vi "Main.vi"(11 "Module Admin":refnum<class "Delacor_lib_QMH_Cloneable Module Admin.lvclass">) -> ()   [LabVIEW 2025, in "Stepper.lvlib"]
doc: "This template is based off of the Queued Message Handler design pattern and the Queued Message Handler project template that ships with LabVIEW.\n\nThe main difference is that the queue is private to this module and communication between modules is performed via Broadcast and Request events.\n\nRequest events are wrapped in public API methods and are handled in the Event Handling Loop (EHL) of this VI. Any module can register for Broadcast events sent by this module. The EHL generates messages based on user interface actions.\n\nThe Message Handling Loop (MHL) processes messages generated by the EHL, or by other messages. The messages are string values, so new messages can be added easily to the Message Cases case structure in the MHL. Each message cluster can also provide an optional value for Message Data, which is a variant that can be converted to whatever message-specific data is required.\n_____\nBased on DQMH Dev Tools: Project Template 7.1.2.1547."
uses:
  Stepper.lvlib
  <vilib>/Delacor/Delacor QMH/Libraries/Cloneable Module Admin_class/Delacor_lib_QMH_Cloneable Module Admin.lvclass
  C:/Program Files/National Instruments/LabVIEW 2025/vi.lib/Delacor/Delacor QMH/Libraries/Module Admin_class/Delacor_lib_QMH_Module Admin.lvclass
  Module Data--cluster.ctl
  Classes/Stepper/Stepper.lvclass
  <vilib>/Delacor/Delacor QMH/Libraries/Message Queue_class/Delacor_lib_QMH_Message Queue.lvclass/Delacor_lib_QMH_Message Queue.ctl
  <vilib>/Delacor/Delacor QMH/Libraries/Cloneable Module Admin_class/Delacor_lib_QMH_Cloneable Module Admin.lvclass/Delacor_lib_QMH_Cloneable Module Admin.ctl
  Stop Argument--cluster.ctl
  <vilib>/Delacor/Delacor QMH/Libraries/Module Admin_class/Delacor_lib_QMH_Module Admin.lvclass/Delacor_lib_QMH_Module Admin.ctl
  close Argument--cluster.ctl
  close (Reply Payload)--cluster.ctl
  init driver Argument--cluster.ctl
  init driver (Reply Payload)--cluster.ctl
  Clear Motor Error Argument--cluster.ctl
  Clear Motor Error (Reply Payload)--cluster.ctl
  read config Argument--cluster.ctl
  read config (Reply Payload)--cluster.ctl
  Read Angle Argument--cluster.ctl
  Read Angle (Reply Payload)--cluster.ctl
  Jog Argument--cluster.ctl
  Jog (Reply Payload)--cluster.ctl
  Go To Angle Argument--cluster.ctl
  Go To Angle (Reply Payload)--cluster.ctl
  <vilib>/Utility/miscctls.llb/LVPointTypeDef.ctl
  <vilib>/Delacor/Delacor QMH/Libraries/Message Queue_class/Delacor_lib_QMH_Enqueue Message (Single).vi
  <vilib>/Delacor/Delacor QMH/Libraries/Cloneable Module Admin_class/Delacor_lib_QMH_Get Module ID.vi
  <vilib>/Delacor/Delacor QMH/Libraries/Module Admin_class/Delacor_lib_QMH_Get External Launch.vi
  <vilib>/Delacor/Delacor QMH/Libraries/Message Queue_class/Delacor_lib_QMH_Message Queue.lvclass
panel:
  out "error out":errorcluster
  out "Status":string
  in  "Simulate EHL Error":bool
  in  "Simulate MHL Error":bool
  # "Other processes communicate with this Module via its Public API (wrappers for its Request Events).\n\nThis Module communicates with other processes via its Broadcast Events.\nAny process that wants to receive these messages can register for this module's Broadcast events."
  # "This template is for the DQMH framework. See the block diagram for more information on how to use this template."
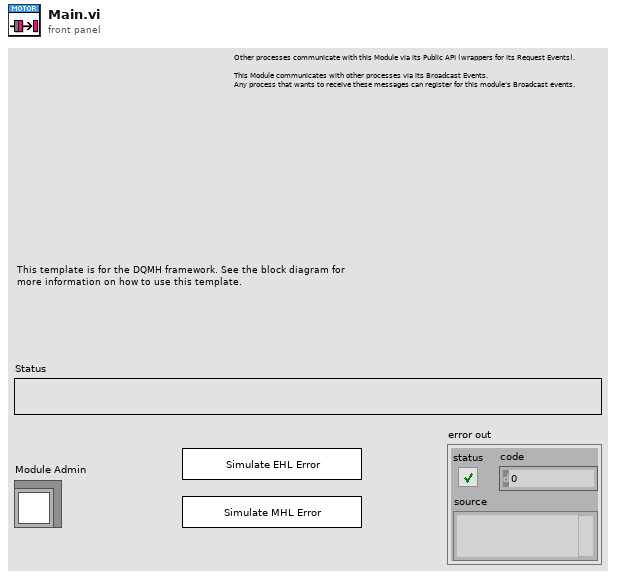
[diagram p1: front panel]
types:
  T1 = typedef "Stepper.lvlib/Request Events--cluster.ctl" = cluster{"Stop Module":refnum<user-event>, "Show Panel":refnum<user-event>, "Hide Panel":refnum<user-event>, "Show Diagram":refnum<user-event>, "Get Module Execution Status":refnum<user-event>, "close":refnum<user-event>, "init":refnum<user-event>, "init driver":refnum<user-event>, "Clear Motor Error":refnum<user-event>, "read config":refnum<user-event>, "Read Angle":refnum<user-event>, "Jog":refnum<user-event>, "Go To Angle":refnum<user-event>}
  T2 = typedef "Stepper.lvlib/Module Data--cluster.ctl" = cluster{"Status":string, "Stepper":refnum<class "Stepper.lvclass">}
  T3 = enum32{"invalid lock state", "Not Locked", "Locked (No Password)", "Password-protected"}
  T4 = typedef "Stepper.lvlib/Stop Argument--cluster.ctl" = cluster{"Module ID":i32, "Origin":string, "Exit via Stop Module Req?":bool, "Wait for Module to stop?":bool}
  T5 = typedef "Stepper.lvlib/close Argument--cluster.ctl" = cluster{"Module ID":i32, "Wait Notifier":refnum<notifier>, "wait for reply":bool}
  T6 = typedef "Stepper.lvlib/init driver Argument--cluster.ctl" = cluster{"Module ID":i32, "Wait Notifier":refnum<notifier>, "wait for reply":bool}
  T7 = typedef "Stepper.lvlib/Clear Motor Error Argument--cluster.ctl" = cluster{"Module ID":i32, "Wait Notifier":refnum<notifier>, "wait for reply":bool}
  T8 = typedef "Stepper.lvlib/read config Argument--cluster.ctl" = cluster{"Module ID":i32, "config file path":path, "Wait Notifier":refnum<notifier>, "wait for reply":bool}
  T9 = typedef "Stepper.lvlib/Read Angle Argument--cluster.ctl" = cluster{"Module ID":i32, "Wait Notifier":refnum<notifier>, "wait for reply":bool}
  T10 = typedef "Stepper.lvlib/Jog Argument--cluster.ctl" = cluster{"Module ID":i32, "CCW? (T)":bool, "[rpm]":u16, "Wait Notifier":refnum<notifier>, "wait for reply":bool}
  T11 = typedef "Stepper.lvlib/Go To Angle Argument--cluster.ctl" = cluster{"Module ID":i32, "Angle":dbl, "Velocity [rpm]":i32, "Pause Time [ms]":i32, "Wait Notifier":refnum<notifier>, "wait for reply":bool}
  T12 = typedef "LVPointTypeDef.ctl" = cluster{"Horizontal":i16, "Vertical":i16}
  T13 = enum32{"Invalid", "Standard", "Closed", "Hidden", "Minimized", "Maximized"}
  T14 = typedef "Stepper.lvlib/close (Reply Payload)--cluster.ctl" = cluster{"Module ID":i32, "error":errorcluster}
  T15 = typedef "Stepper.lvlib/init driver (Reply Payload)--cluster.ctl" = cluster{"Module ID":i32, "error":errorcluster}
  T16 = typedef "Stepper.lvlib/Clear Motor Error (Reply Payload)--cluster.ctl" = cluster{"Module ID":i32, "error":errorcluster}
  T17 = typedef "Stepper.lvlib/read config (Reply Payload)--cluster.ctl" = cluster{"Module ID":i32, "error":errorcluster}
  T18 = typedef "Stepper.lvlib/Read Angle (Reply Payload)--cluster.ctl" = cluster{"Module ID":i32, "Angle":dbl, "error":errorcluster}
  T19 = typedef "Stepper.lvlib/Jog (Reply Payload)--cluster.ctl" = cluster{"Module ID":i32, "Angle":dbl, "error":errorcluster}
  T20 = typedef "Stepper.lvlib/Go To Angle (Reply Payload)--cluster.ctl" = cluster{"Module ID":i32, "Angle":dbl, "error":errorcluster}
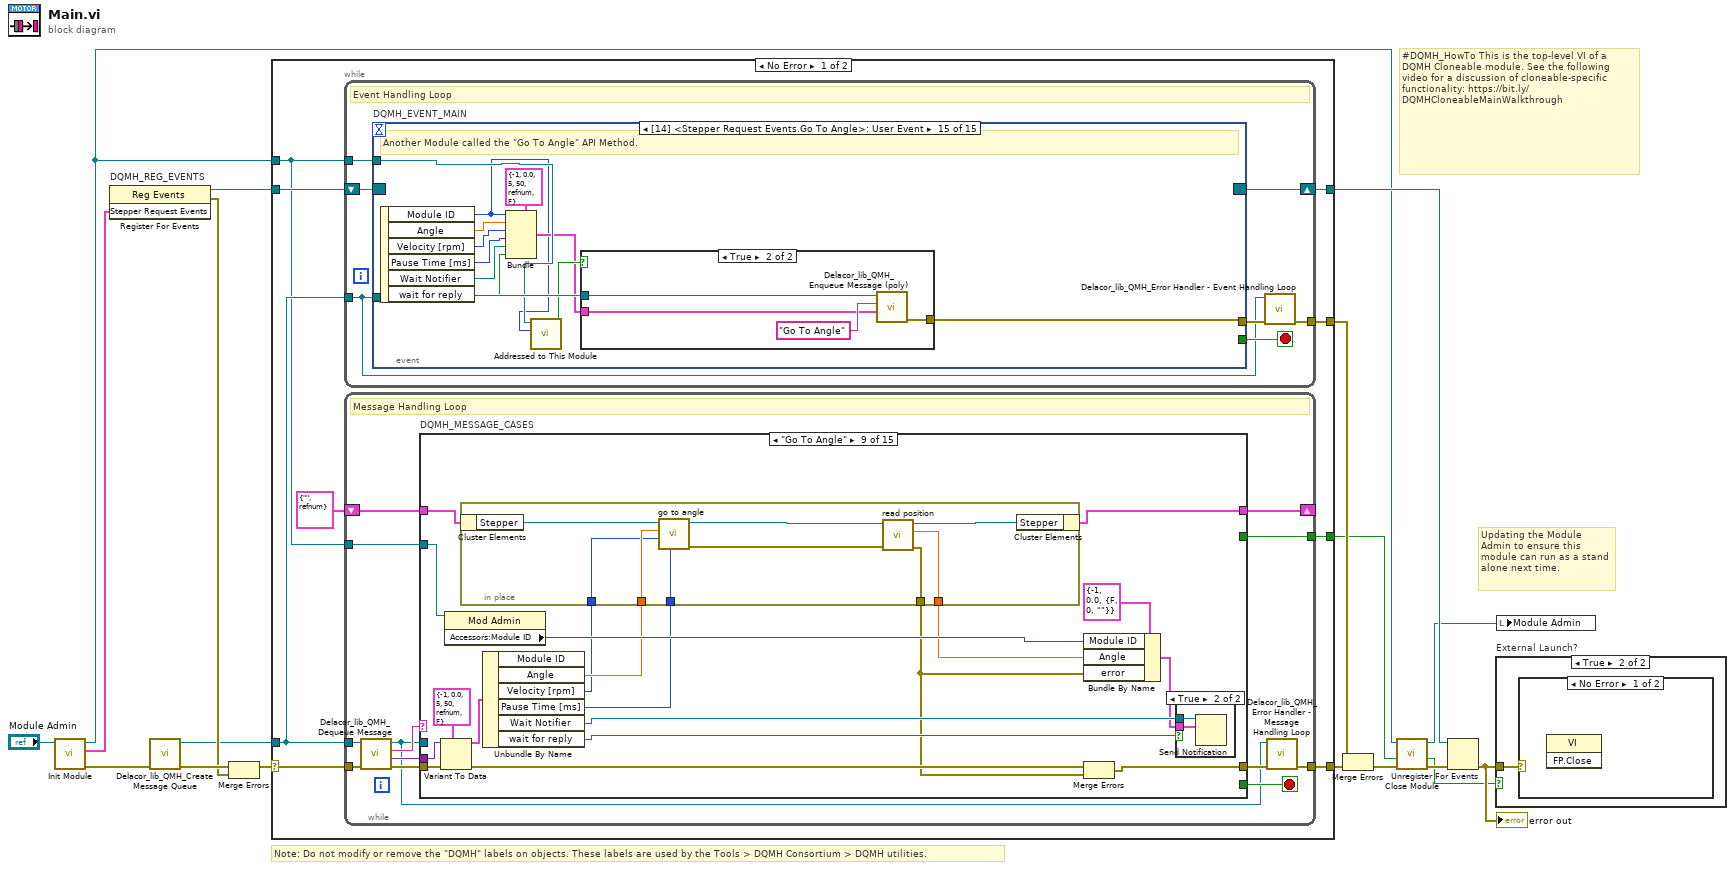
[diagram p0: block diagram]
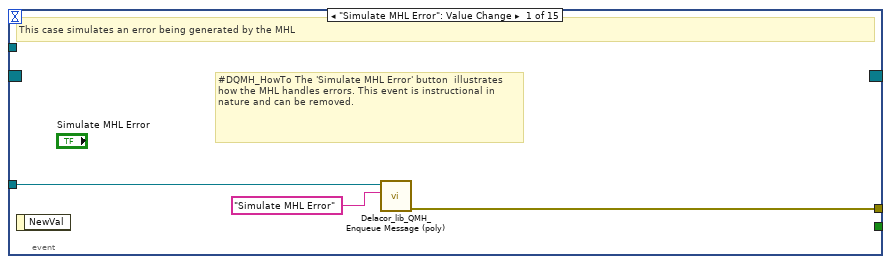
[diagram p2: hidden frame]
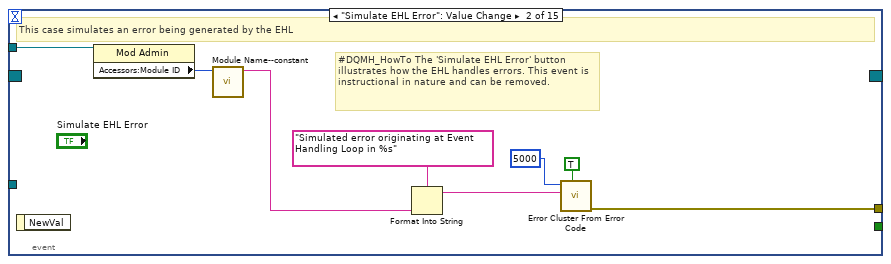
[diagram p3: hidden frame]
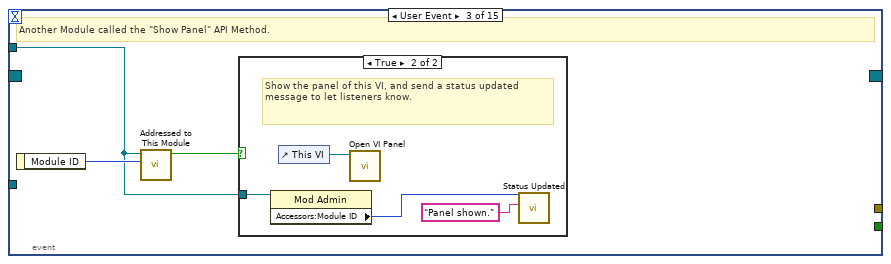
[diagram p4: hidden frame]
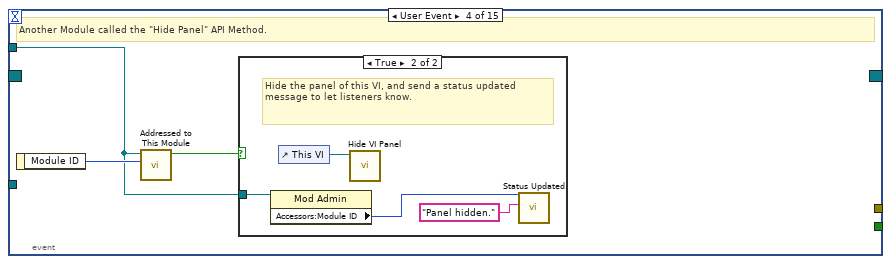
[diagram p6: hidden frame]
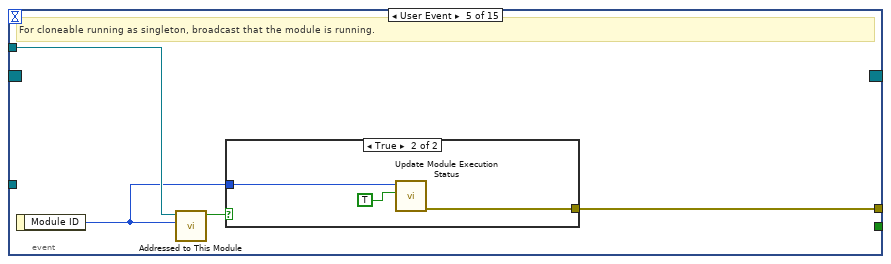
[diagram p8: hidden frame]
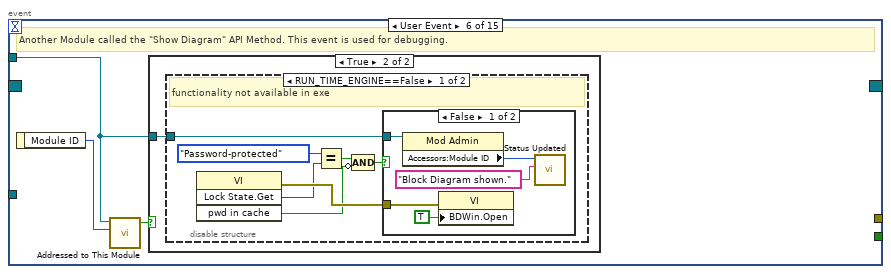
[diagram p10: hidden frame]
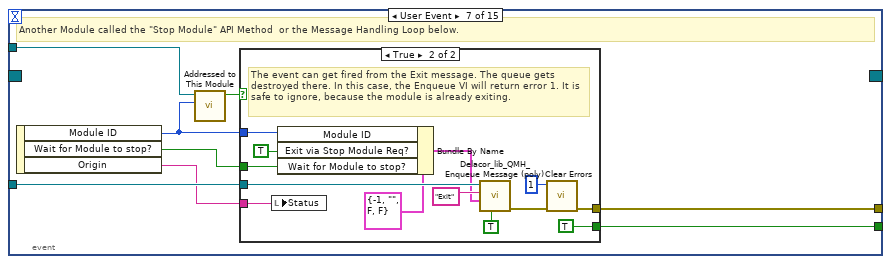
[diagram p14: hidden frame]
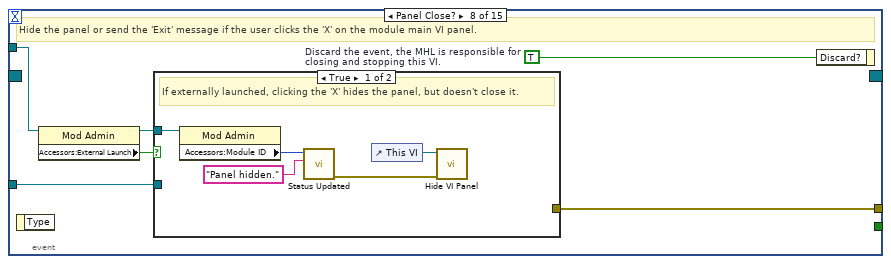
[diagram p16: hidden frame]
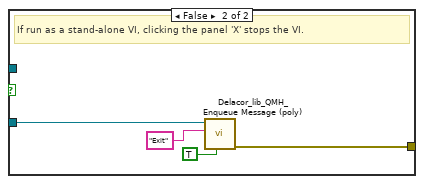
[diagram p17: hidden frame]
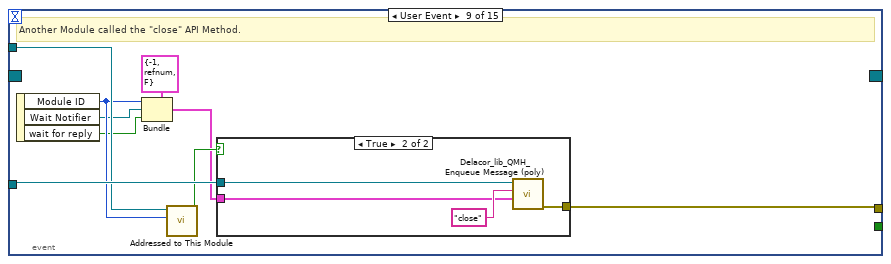
[diagram p18: hidden frame]
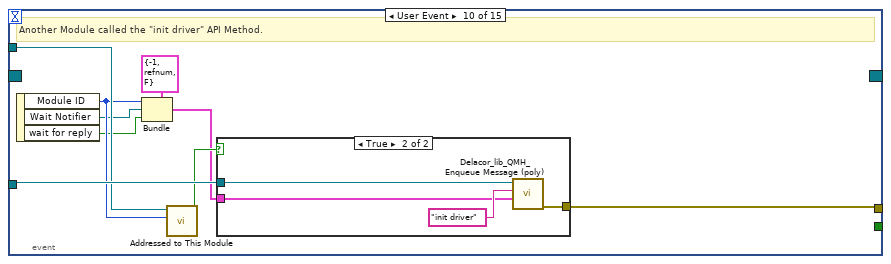
[diagram p20: hidden frame]
diagram:
  # "#DQMH_HowTo This is the top-level VI of a DQMH Cloneable module. See the following video for a discussion of cloneable-specific functionality: https://bit.ly/DQMHCloneableMainWalkthrough"
  # "Note: Do not modify or remove the \"DQMH\" labels on objects. These labels are used by the Tools > DQMH Consortium > DQMH utilities."
  # "Updating the Module Admin to ensure this module can run as a stand alone next time."
  n1 = call "Init Module.vi"("Cloneable Module Admin in"="Module Admin") -> ("error out"=w15:errorcluster, "Stepper Request Events"=w7:T1, "Cloneable Module Admin out"=w4:refnum<class "Delacor_lib_QMH_Cloneable Module Admin.lvclass">)  [unwired: 8 in]
  n2 = register-events "DQMH_REG_EVENTS"(w7) -> (reference out=w8:refnum<event-registration>, error out=w10:errorcluster)  [unwired: 2 in]
  n3 = call <vilib>:"Delacor_lib_QMH_Create Message Queue.vi"("error in"=w15) -> ("error out"=w12:errorcluster, "Message Queue"=w6:refnum<class "Delacor_lib_QMH_Message Queue.lvclass">)  [unwired: 9 in]
  n4 = Merge Errors(w12, w10) -> (w11:errorcluster)
  n5 = case shown="No Error" w11 {
    selector: w11 -> [w25 w489]
    tunnel: [w27 w488] -> w16
    tunnel: [w24 w487] -> w9
    tunnel: w8 -> [w22 w487]
    tunnel: w6 -> [w21 w480]
    tunnel: [w26 _] -> w17
    tunnel: w4 -> [w20 w483]
    tunnel: [w19 _] -> w2
    frame No Error {
      n6 = while {
        tunnel: w21 -> [w28]
        shift-right: [w31] -> w24
        shift-left: w22 -> [w32]
        tunnel: [w33] -> w26
        tunnel: w20 -> [w29]
        stop <- w30 stop-if-true
        # "Event Handling Loop"
        n7 = event "DQMH_EVENT_MAIN" shown="[14] <Stepper Request Events.Go To Angle>: User Event" {
          selector: w32 -> [_ _ _ _ _ _ _ _ _ _ _ _ _ _ _]
          dyn-events: [_ _ _ _ _ _ _ _ _ _ _ _ _ _ _] -> w31
          timeout: _ -> [_ _ _ _ _ _ _ _ _ _ _ _ _ _ _]
          tunnel: [_ _ _ _ _ _ w86 _ _ _ _ _ _ _ _] -> w30
          tunnel: w28 -> [w36 _ _ _ _ _ w89 w106 w127 w140 w153 w167 w180 w195 w211]
          tunnel: [w37 w45 _ _ w63 _ w90 w109 w119 w132 w145 w158 w172 w185 w200] -> w34
          tunnel: w29 -> [_ w44 w46 w53 w61 w67 w88 w107 w125 w138 w151 w165 w178 w193 w209]
          event "Simulate MHL Error": Value Change {
            # "#DQMH_HowTo The 'Simulate MHL Error' button  illustrates how the MHL handles errors. This event is instructional in nature and can be removed."
            # "This case simulates an error being generated by the MHL"
            n8 = event-data() -> ()  [unwired: 1 in, 1 out]
            n9 = call-poly <vilib>:"Delacor_lib_QMH_Enqueue Message (poly).vi"("Message"="Simulate MHL Error", "Message Queue in"=w36) -> ("error out"=w37:errorcluster)  [unwired: 8 in, 1 out]
          }
          event "Simulate EHL Error": Value Change {
            # "#DQMH_HowTo The 'Simulate EHL Error' button  illustrates how the EHL handles errors. This event is instructional in nature and can be removed."
            # "This case simulates an error being generated by the EHL"
            n10 = event-data() -> ()  [unwired: 1 in, 1 out]
            n11 = property on="Property Node" class="Mod Admin"(reference=w44) -> ("Accessors:Module ID"=w43:i32)  [unwired: 1 in, 2 out]
            n12 = call "Module Name--constant.vi"("Module ID"=w43) -> ("Module Name"=w38:string)  [unwired: 10 in]
            n13 = Format Into String(format string="Simulated error originating at Event Handling Loop in %s", w38) -> (resulting string=w41:string)  [unwired: 2 in, 1 out]
            n14 = call <vilib>:"Error Cluster From Error Code.vi"("show call chain? (False)"=TRUE, "error message (\"\")"=w41, "error code (0)"=5000) -> ("error out"=w45:errorcluster)  [unwired: 6 in]
          }
          event User Event {
            # "Another Module called the \"Show Panel\" API Method."
            n15 = event-data() -> ("Module ID"=w47:i32)  [unwired: 1 in]
            n16 = call "Addressed to This Module.vi"("Module ID from Argument"=w47, "Module Admin"=w46) -> ("Addressed to this instance?"=w48:bool)  [unwired: 8 in, 1 out]
            n17 = case shown="True" w48 {
              tunnel: w46 -> [_ w50]
              frame False {
              }
              frame True {
                # "Show the panel of this VI, and send a status updated message to let listeners know."
                n18 = property on="Property Node" class="Mod Admin"(reference=w50) -> ("Accessors:Module ID"=w49:i32)  [unwired: 1 in, 2 out]
                n19 = control-ref of="This VI"() -> (w52:refnum<vi>)
                n20 = call "Open VI Panel.vi"("VI"=w52) -> ()  [unwired: 10 in, 1 out]
                n21 = call "Status Updated.vi"("Status"="Panel shown." ("format string"), "Module ID"=w49) -> ()  [unwired: 9 in, 1 out]
              }
            }
          }
          event User Event {
            # "Another Module called the \"Hide Panel\" API Method."
            n22 = event-data() -> ("Module ID"=w54:i32)  [unwired: 1 in]
            n23 = call "Addressed to This Module.vi"("Module ID from Argument"=w54, "Module Admin"=w53) -> ("Addressed to this instance?"=w55:bool)  [unwired: 8 in, 1 out]
            n24 = case shown="True" w55 {
              tunnel: w53 -> [_ w57]
              frame False {
              }
              frame True {
                # "Hide the panel of this VI, and send a status updated message to let listeners know."
                n25 = property on="Property Node" class="Mod Admin"(reference=w57) -> ("Accessors:Module ID"=w56:i32)  [unwired: 1 in, 2 out]
                n26 = control-ref of="This VI"() -> (w59:refnum<vi>)
                n27 = call "Hide VI Panel.vi"("VI"=w59) -> ()  [unwired: 10 in, 1 out]
                n28 = call "Status Updated.vi"("Status"="Panel hidden." ("format string"), "Module ID"=w56) -> ()  [unwired: 9 in, 1 out]
              }
            }
          }
          event User Event {
            # "For cloneable running as singleton, broadcast that the module is running."
            n29 = event-data() -> ("Module ID"=w60:i32)  [unwired: 1 in]
            n30 = call "Addressed to This Module.vi"("Module ID from Argument"=w60, "Module Admin"=w61) -> ("Addressed to this instance?"=w62:bool)  [unwired: 8 in, 1 out]
            n31 = case shown="True" w62 {
              tunnel: [_ w66] -> w63
              tunnel: w60 -> [_ w65]
              frame False {
              }
              frame True {
                n32 = call "Update Module Execution Status.vi"("Running?"=TRUE, "Module ID"=w65) -> ("error out"=w66:errorcluster)  [unwired: 9 in]
              }
            }
          }
          event User Event {
            # "Another Module called the \"Show Diagram\" API Method. This event is used for debugging."
            n33 = event-data() -> ("Module ID"=w68:i32)  [unwired: 1 in]
            n34 = call "Addressed to This Module.vi"("Module ID from Argument"=w68, "Module Admin"=w67) -> ("Addressed to this instance?"=w69:bool)  [unwired: 8 in, 1 out]
            n35 = case shown="True" w69 {
              tunnel: w67 -> [_ w70]
              frame False {
              }
              frame True {
                n36 = disable-structure shown="RUN_TIME_ENGINE==False" {
                  disable-tunnel: w70 -> [w71 _]
                  frame condition #0 (active) {
                    # "functionality not available in exe"
                    n37 = invoke on="Invoke Node" class="VI" method="Lock State.Get"() -> (error out=w77:errorcluster, "Get Lock State"=w76:T3, "pwd in cache"=w73:bool)  [unwired: 4 in, 1 out]
                    n38 = Equal?(x=T3."Password-protected", y=w76) -> (x = y?=w74:bool)
                    n39 = Compound Arithmetic op=AND(w74, invert w73) -> (w72:bool)
                    n40 = case shown="False" w72 {
                      tunnel: w77 -> [w82 _]
                      tunnel: w71 -> [w79 _]
                      frame False {
                        n41 = property on="Property Node" class="Mod Admin"(reference=w79) -> ("Accessors:Module ID"=w78:i32)  [unwired: 1 in, 2 out]
                        n42 = property on="Property Node" class="VI"(error in=w82, "BDWin.Open"=TRUE ("Block Diagram Window:Open")) -> ()  [unwired: 1 in, 2 out]
                        n43 = call "Status Updated.vi"("Status"="Block Diagram shown." ("format string"), "Module ID"=w78) -> ()  [unwired: 9 in, 1 out]
                      }
                      frame True {
                        # "Password-protected VI, and the password is not in the cache. Do not show the diagram."
                      }
                    }
                  }
                  frame condition #1 {
                  }
                }
              }
            }
          }
          event User Event {
            # "Another Module called the \"Stop Module\" API Method  or the Message Handling Loop below."
            n44 = event-data() -> ("Module ID"=w84:i32, "Wait for Module to stop?"=w85:bool, "Origin"=w83:string)  [unwired: 1 in]
            n45 = call "Addressed to This Module.vi"("Module ID from Argument"=w84, "Module Admin"=w88) -> ("Addressed to this instance?"=w87:bool)  [unwired: 8 in, 1 out]
            n46 = case shown="True" w87 {
              tunnel: [_ w102] -> w90
              tunnel: w89 -> [_ w98]
              tunnel: [_ TRUE] -> w86
              tunnel: w85 -> [_ w93]
              tunnel: w84 -> [_ w95]
              tunnel: w83 -> [_ w91]
              frame False {
              }
              frame True {
                # "The event can get fired from the Exit message. The queue gets destroyed there. In this case, the Enqueue VI will return error 1. It is safe to ignore, because the module is already exiting."
                n47 = local write "Status"(w91) -> ()
                n48 = Bundle By Name(cluster=T4 {"Module ID"=-1, "Origin"="", "Exit via Stop Module Req?"=FALSE, "Wait for Module to stop?"=FALSE} ("Stop Argument"), "Module ID"=w95, "Exit via Stop Module Req?"=TRUE, "Wait for Module to stop?"=w93) -> (w92:T4)
                n49 = call-poly <vilib>:"Delacor_lib_QMH_Enqueue Message (poly).vi"("Priority Message? (F)"=TRUE, "Message Data"=w92, "Message"="Exit", "Message Queue in"=w98) -> ("error out"=w103:errorcluster)  [unwired: 6 in, 1 out]
                n50 = call <vilib>:"Clear Errors.vi"("error in (no error)"=w103, "specific error code to clear (0: all)"=1) -> ("error out"=w102:errorcluster)  [unwired: 4 in, 1 out]
              }
            }
          }
          event Panel Close? {
            w108 = TRUE  # Discard the event, the MHL is responsible for closing and stopping this VI.
            # "Hide the panel or send the 'Exit' message if the user clicks the 'X' on the module main VI panel."
            n51 = event-data() -> ()  [unwired: 1 in, 1 out]
            n52 = property on="Property Node" class="Mod Admin"(reference=w107) -> (reference out=w104:refnum<class "Delacor_lib_QMH_Cloneable Module Admin.lvclass">, "Accessors:External Launch"=w105:bool)  [unwired: 1 in, 1 out]
            n53 = case shown="True" w105 {
              tunnel: w106 -> [_ w117]
              tunnel: [_ w118] -> w109
              tunnel: w104 -> [w112 _]
              frame True {
                # "If externally launched, clicking the 'X' hides the panel, but doesn't close it."
                n54 = property on="Property Node" class="Mod Admin"(reference=w112) -> ("Accessors:Module ID"=w111:i32)  [unwired: 1 in, 2 out]
                n55 = call "Status Updated.vi"("Status"="Panel hidden." ("format string"), "Module ID"=w111) -> ("error out"=w110:errorcluster)  [unwired: 9 in]
                n56 = control-ref of="This VI"() -> (w114:refnum<vi>)
                n57 = call "Hide VI Panel.vi"("error in"=w110, "VI"=w114) -> ()  [unwired: 9 in, 1 out]
              }
              frame False {
                # "If run as a stand-alone VI, clicking the panel 'X' stops the VI."
                n58 = call-poly <vilib>:"Delacor_lib_QMH_Enqueue Message (poly).vi"("Priority Message? (F)"=TRUE, "Message"="Exit", "Message Queue in"=w117) -> ("error out"=w118:errorcluster)  [unwired: 7 in, 1 out]
              }
            }
            n59 = event-data ("Event Filter Node")("Discard?"=w108) -> ()  [unwired: 1 in, 1 out]
          }
          event User Event {
            # "Another Module called the \"close\" API Method."
            n60 = event-data() -> ("Module ID"=w122:i32, "Wait Notifier"=w121:refnum<notifier>, "wait for reply"=w120:bool)  [unwired: 1 in]
            n61 = Bundle(cluster=T5 {"Module ID"=-1, "Wait Notifier"=refnum, "wait for reply"=FALSE} ("close Argument"), "Module ID"=w122, "Wait Notifier"=w121, "wait for reply"=w120) -> (w123:T5)
            n62 = call "Addressed to This Module.vi"("Module ID from Argument"=w122, "Module Admin"=w125) -> ("Addressed to this instance?"=w126:bool)  [unwired: 8 in, 1 out]
            n63 = case shown="True" w126 {
              tunnel: w127 -> [_ w131]
              tunnel: w123 -> [_ w129]
              tunnel: [_ w128] -> w119
              frame False {
              }
              frame True {
                n64 = call-poly <vilib>:"Delacor_lib_QMH_Enqueue Message (poly).vi"("Message Data"=w129, "Message"="close", "Message Queue in"=w131) -> ("error out"=w128:errorcluster)  [unwired: 7 in, 1 out]
              }
            }
          }
          event User Event {
            # "Another Module called the \"init driver\" API Method."
            n65 = event-data() -> ("Module ID"=w135:i32, "Wait Notifier"=w134:refnum<notifier>, "wait for reply"=w133:bool)  [unwired: 1 in]
            n66 = Bundle(cluster=T6 {"Module ID"=-1, "Wait Notifier"=refnum, "wait for reply"=FALSE} ("init driver Argument"), "Module ID"=w135, "Wait Notifier"=w134, "wait for reply"=w133) -> (w136:T6)
            n67 = call "Addressed to This Module.vi"("Module ID from Argument"=w135, "Module Admin"=w138) -> ("Addressed to this instance?"=w139:bool)  [unwired: 8 in, 1 out]
            n68 = case shown="True" w139 {
              tunnel: w140 -> [_ w144]
              tunnel: w136 -> [_ w142]
              tunnel: [_ w141] -> w132
              frame False {
              }
              frame True {
                n69 = call-poly <vilib>:"Delacor_lib_QMH_Enqueue Message (poly).vi"("Message Data"=w142, "Message"="init driver", "Message Queue in"=w144) -> ("error out"=w141:errorcluster)  [unwired: 7 in, 1 out]
              }
            }
          }
          event User Event {
            # "Another Module called the \"Clear Motor Error\" API Method."
            n70 = event-data() -> ("Module ID"=w148:i32, "Wait Notifier"=w147:refnum<notifier>, "wait for reply"=w146:bool)  [unwired: 1 in]
            n71 = Bundle(cluster=T7 {"Module ID"=-1, "Wait Notifier"=refnum, "wait for reply"=FALSE} ("Clear Motor Error Argument"), "Module ID"=w148, "Wait Notifier"=w147, "wait for reply"=w146) -> (w149:T7)
            n72 = call "Addressed to This Module.vi"("Module ID from Argument"=w148, "Module Admin"=w151) -> ("Addressed to this instance?"=w152:bool)  [unwired: 8 in, 1 out]
            n73 = case shown="True" w152 {
              tunnel: w153 -> [_ w157]
              tunnel: w149 -> [_ w155]
              tunnel: [_ w154] -> w145
              frame False {
              }
              frame True {
                n74 = call-poly <vilib>:"Delacor_lib_QMH_Enqueue Message (poly).vi"("Message Data"=w155, "Message"="Clear Motor Error", "Message Queue in"=w157) -> ("error out"=w154:errorcluster)  [unwired: 7 in, 1 out]
              }
            }
          }
          event User Event {
            # "Another Module called the \"read config\" API Method."
            n75 = event-data() -> ("Module ID"=w162:i32, "config file path"=w161:path, "Wait Notifier"=w160:refnum<notifier>, "wait for reply"=w159:bool)  [unwired: 1 in]
            n76 = Bundle(cluster=T8 {"Module ID"=-1, "config file path"=path "", "Wait Notifier"=refnum, "wait for reply"=FALSE} ("read config Argument"), "Module ID"=w162, "config file path"=w161, "Wait Notifier"=w160, "wait for reply"=w159) -> (w163:T8)
            n77 = call "Addressed to This Module.vi"("Module ID from Argument"=w162, "Module Admin"=w165) -> ("Addressed to this instance?"=w166:bool)  [unwired: 8 in, 1 out]
            n78 = case shown="True" w166 {
              tunnel: w167 -> [_ w171]
              tunnel: w163 -> [_ w169]
              tunnel: [_ w168] -> w158
              frame False {
              }
              frame True {
                n79 = call-poly <vilib>:"Delacor_lib_QMH_Enqueue Message (poly).vi"("Message Data"=w169, "Message"="read config", "Message Queue in"=w171) -> ("error out"=w168:errorcluster)  [unwired: 7 in, 1 out]
              }
            }
          }
          event User Event {
            # "Another Module called the \"Read Angle\" API Method."
            n80 = event-data() -> ("Module ID"=w175:i32, "Wait Notifier"=w174:refnum<notifier>, "wait for reply"=w173:bool)  [unwired: 1 in]
            n81 = Bundle(cluster=T9 {"Module ID"=-1, "Wait Notifier"=refnum, "wait for reply"=FALSE} ("Read Angle Argument"), "Module ID"=w175, "Wait Notifier"=w174, "wait for reply"=w173) -> (w176:T9)
            n82 = call "Addressed to This Module.vi"("Module ID from Argument"=w175, "Module Admin"=w178) -> ("Addressed to this instance?"=w179:bool)  [unwired: 8 in, 1 out]
            n83 = case shown="True" w179 {
              tunnel: w180 -> [_ w184]
              tunnel: w176 -> [_ w182]
              tunnel: [_ w181] -> w172
              frame False {
              }
              frame True {
                n84 = call-poly <vilib>:"Delacor_lib_QMH_Enqueue Message (poly).vi"("Message Data"=w182, "Message"="Read Angle", "Message Queue in"=w184) -> ("error out"=w181:errorcluster)  [unwired: 7 in, 1 out]
              }
            }
          }
          event User Event {
            # "Another Module called the \"Jog\" API Method."
            n85 = event-data() -> ("Module ID"=w190:i32, "CCW? (T)"=w189:bool, "[rpm]"=w188:u16, "Wait Notifier"=w187:refnum<notifier>, "wait for reply"=w186:bool)  [unwired: 1 in]
            n86 = Bundle(cluster=T10 {"Module ID"=-1, "CCW? (T)"=TRUE, "[rpm]"=60, "Wait Notifier"=refnum, "wait for reply"=FALSE} ("Jog Argument"), "Module ID"=w190, "CCW? (T)"=w189, "[rpm]"=w188, "Wait Notifier"=w187, "wait for reply"=w186) -> (w191:T10)
            n87 = call "Addressed to This Module.vi"("Module ID from Argument"=w190, "Module Admin"=w193) -> ("Addressed to this instance?"=w194:bool)  [unwired: 8 in, 1 out]
            n88 = case shown="True" w194 {
              tunnel: w195 -> [_ w199]
              tunnel: w191 -> [_ w197]
              tunnel: [_ w196] -> w185
              frame False {
              }
              frame True {
                n89 = call-poly <vilib>:"Delacor_lib_QMH_Enqueue Message (poly).vi"("Message Data"=w197, "Message"="Jog", "Message Queue in"=w199) -> ("error out"=w196:errorcluster)  [unwired: 7 in, 1 out]
              }
            }
          }
          event User Event {
            # "Another Module called the \"Go To Angle\" API Method."
            n90 = event-data() -> ("Module ID"=w206:i32, "Angle"=w205:dbl, "Velocity [rpm]"=w204:i32, "Pause Time [ms]"=w203:i32, "Wait Notifier"=w202:refnum<notifier>, "wait for reply"=w201:bool)  [unwired: 1 in]
            n91 = Bundle(cluster=T11 {"Module ID"=-1, "Angle"=0.0, "Velocity [rpm]"=5, "Pause Time [ms]"=50, "Wait Notifier"=refnum, "wait for reply"=FALSE} ("Go To Angle Argument"), "Module ID"=w206, "Angle"=w205, "Velocity [rpm]"=w204, "Pause Time [ms]"=w203, "Wait Notifier"=w202, "wait for reply"=w201) -> (w207:T11)
            n92 = call "Addressed to This Module.vi"("Module ID from Argument"=w206, "Module Admin"=w209) -> ("Addressed to this instance?"=w210:bool)  [unwired: 8 in, 1 out]
            n93 = case shown="True" w210 {
              tunnel: w211 -> [_ w215]
              tunnel: w207 -> [_ w213]
              tunnel: [_ w212] -> w200
              frame False {
              }
              frame True {
                n94 = call-poly <vilib>:"Delacor_lib_QMH_Enqueue Message (poly).vi"("Message Data"=w213, "Message"="Go To Angle", "Message Queue in"=w215) -> ("error out"=w212:errorcluster)  [unwired: 7 in, 1 out]
              }
            }
          }
        }
        n95 = call-dynamic "Delacor_lib_QMH_Error Handler - Event Handling Loop.vi"("error in"=w34, "Message Queue in"=w28) -> ("dup error in"=w33:errorcluster)  [unwired: 8 in, 1 out]
      }
      n96 = while {
        tunnel: w21 -> [w216]
        shift-right: [w223] -> _
        shift-left: T2 {"Status"="", "Stepper"=refnum} ("Data Cluster") -> [w224]
        tunnel: w25 -> [w227]
        tunnel: [w225] -> w27
        tunnel: w20 -> [w218]
        tunnel: [w217] -> w19
        stop <- w222 stop-if-true
        # "Message Handling Loop"
        n97 = call-dynamic "Delacor_lib_QMH_Dequeue Message.vi"("error in"=w227, "Message Queue in"=w216) -> ("error out"=w226:errorcluster, "Message Data"=w220:variant, "Message"=w221:string, "Message Queue out"=w219:refnum<class "Delacor_lib_QMH_Message Queue.lvclass">)  [unwired: 6 in]
        n98 = case "DQMH_MESSAGE_CASES" shown="\"Go To Angle\"" w221 {
          selector: w221 -> [_ _ _ _ _ _ _ _ _ _ _ _ _ _ w469]
          tunnel: w219 -> [_ _ _ _ _ _ _ _ _ _ _ w424 _ w461 _]
          tunnel: w226 -> [w247 w251 w266 w286 w306 w327 w349 w373 w405 w419 w421 w433 w450 w467 w478]
          tunnel: [w245 w251 w257 w277 w297 w318 w340 w364 w396 w418 w421 w429 w449 w462 w479] -> w228
          tunnel: w224 -> [w238 w250 w254 w274 w294 w315 w337 w361 w393 w417 w420 w428 w447 w460 w476]
          tunnel: [w237 w250 w252 w273 w292 w312 w334 w360 w392 w417 w420 w428 w447 w460 w476] -> w223
          tunnel: [_ _ _ _ _ _ _ _ _ _ _ _ _ w459 _] -> w222
          tunnel: w220 -> [_ _ w264 w284 w304 w325 w347 w371 w403 _ _ w427 _ w457 _]
          tunnel: w218 -> [w233 _ w255 w275 w295 w316 w338 w362 w394 _ _ w426 w445 w452 w475]
          tunnel: [_ _ _ _ _ _ _ _ _ _ _ _ _ w455 _] -> w217
          frame "Initialize" {
            w230 = "Initial Message" ("Initial Message")
            # "#DQMH_CodeNeeded - Initialize the appearance of the front panel."
            # "#DQMH_CodeNeeded - Initialize your state data here."
            # "Initialize - Any operation that needs to be done before the module can receive messages. Synchronize Caller Events.vi will inform Start Module.vi that the module has launched and is ready to receive messages. Module Did Init.vi will broadcast that the module initialized."
            n99 = call "Synchronize Caller Events.vi"("error in"=w247, "Module Admin"=w233) -> ("error out"=w246:errorcluster, "Module Admin out"=w232:refnum<class "Delacor_lib_QMH_Cloneable Module Admin.lvclass">)  [unwired: 8 in]
            n100 = property on="Property Node" class="Mod Admin"(reference=w232) -> ("Accessors:Module ID"=w229:i32, "Accessors:External Launch"=w234:bool)  [unwired: 1 in, 2 out]
            n101 = call "Module Name--constant.vi"("Module ID"=w229) -> ("Module Name"=w242:string)  [unwired: 10 in]
            n102 = property on="Property Node" class="VI"("Front Panel.Title"=w242) -> (reference out=w244:refnum<vi>, error out=w249:errorcluster)  [unwired: 2 in]
            n103 = Select(t=T13."Hidden" ("State"), s=w234, f=T13."Standard" ("State")) -> (s? t:f=w239:T13)
            n104 = invoke on="Invoke Node" class="VI" method="FP.Open"(reference=w244, error in=w249, "State"=w239) -> (reference out=w243:refnum<vi>, error out=w248:errorcluster)  [unwired: 2 in, 3 out]
            n105 = Bundle By Name(cluster=w238, "Status"=w230) -> (w237:T2)
            n106 = invoke on="Invoke Node" class="VI" method="FP.Center"(reference=w243, error in=w248) -> ()  [unwired: 1 in, 3 out]
            n107 = property on="Pane" class="Pane"("Origin"=T12 {"Horizontal"=0, "Vertical"=0}) -> ()  [unwired: 2 in, 2 out]
            n108 = call "Module Name--constant.vi"("Module ID"=w229) -> ("Module Name"=w235:string)  [unwired: 10 in]
            n109 = call "Module Did Init.vi"("error in"=w246, "Initialized?"=TRUE, "Origin"=w235, "Module ID"=w229) -> ("error out"=w245:errorcluster)  [unwired: 7 in]
            "Status" <- w230
          }
          frame "---Module Specific---" {
            # "Separator -- The following cases handle messages specific to this Module."
          }
          frame "close" {
            # "closes Modbus Master Instance"
            n110 = property class="Mod Admin"(reference=w255) -> ("Accessors:Module ID"=w256:i32)  [unwired: 1 in, 2 out]
            n111 = Variant To Data(error in=w266, type=T5 {"Module ID"=-1, "Wait Notifier"=refnum, "wait for reply"=FALSE} ("close Argument"), Variant=w264) -> (data=w262:T5, error out=w265:errorcluster)
            n112 = in-place {
              in-place-border: [w267] -> w253
              n113 = in-place-cluster #1(w254) -> ("Stepper"=w269:refnum<class "Stepper.lvclass">)
              n114 = call-dynamic "close.vi"("Stepper in"=w269) -> ("error out"=w267:errorcluster, "Stepper out"=w268:refnum<class "Stepper.lvclass">)  [unwired: 9 in]
              n115 = in-place-cluster #1("Stepper"=w268) -> (w252:T2)
            }
            n116 = Unbundle By Name(w262) -> ("Wait Notifier"=w261:refnum<notifier>, "wait for reply"=w260:bool)  [unwired: 1 out]
            n117 = Bundle By Name(cluster=T14 {"Module ID"=-1, "error"={"status"=FALSE, "code"=0, "source"=""}} ("close (Reply Payload)"), "Module ID"=w256, "error"=w253) -> (w259:T14)
            n118 = Merge Errors(w265, w253) -> (w257:errorcluster)
            n119 = case "DQMH_FIRE_NOTIFIER" shown="True" w260 {
              tunnel: w261 -> [_ w271]
              tunnel: w259 -> [_ w270]
              frame False {
              }
              frame True {
                n120 = Send Notification(notification=w270, notifier=w271) -> ()  [unwired: 1 in, 2 out]
              }
            }
          }
          frame "init driver" {
            # "Initializes stepper driver for Modbus RTU communication."
            n121 = Variant To Data(error in=w286, type=T6 {"Module ID"=-1, "Wait Notifier"=refnum, "wait for reply"=FALSE} ("init driver Argument"), Variant=w284) -> (data=w282:T6, error out=w285:errorcluster)
            n122 = property class="Mod Admin"(reference=w275) -> ("Accessors:Module ID"=w276:i32)  [unwired: 1 in, 2 out]
            n123 = Unbundle By Name(w282) -> ("Wait Notifier"=w281:refnum<notifier>, "wait for reply"=w280:bool)  [unwired: 1 out]
            n124 = in-place {
              in-place-border: [w287] -> w272
              n125 = in-place-cluster #2(w274) -> ("Stepper"=w289:refnum<class "Stepper.lvclass">)
              n126 = call-dynamic "init.vi"("Stepper in"=w289) -> ("error out"=w287:errorcluster, "Stepper out"=w288:refnum<class "Stepper.lvclass">)  [unwired: 9 in]
              n127 = in-place-cluster #2("Stepper"=w288) -> (w273:T2)
            }
            n128 = Bundle By Name(cluster=T15 {"Module ID"=-1, "error"={"status"=FALSE, "code"=0, "source"=""}} ("init driver (Reply Payload)"), "Module ID"=w276, "error"=w272) -> (w279:T15)
            n129 = Merge Errors(w285, w272) -> (w277:errorcluster)
            n130 = case "DQMH_FIRE_NOTIFIER" shown="True" w280 {
              tunnel: w281 -> [_ w291]
              tunnel: w279 -> [_ w290]
              frame False {
              }
              frame True {
                n131 = Send Notification(notification=w290, notifier=w291) -> ()  [unwired: 1 in, 2 out]
              }
            }
          }
          frame "Clear Motor Error" {
            # "Clear Stepper Driver Error"
            n132 = Variant To Data(error in=w306, type=T7 {"Module ID"=-1, "Wait Notifier"=refnum, "wait for reply"=FALSE} ("Clear Motor Error Argument"), Variant=w304) -> (data=w302:T7, error out=w305:errorcluster)
            n133 = property class="Mod Admin"(reference=w295) -> ("Accessors:Module ID"=w296:i32)  [unwired: 1 in, 2 out]
            n134 = in-place {
              in-place-border: [w307] -> w293
              n135 = in-place-cluster #3(w294) -> ("Stepper"=w309:refnum<class "Stepper.lvclass">)
              n136 = call-dynamic "clear motor error.vi"("Stepper in"=w309) -> ("error out"=w307:errorcluster, "Stepper out"=w308:refnum<class "Stepper.lvclass">)  [unwired: 9 in]
              n137 = in-place-cluster #3("Stepper"=w308) -> (w292:T2)
            }
            n138 = Unbundle By Name(w302) -> ("Wait Notifier"=w301:refnum<notifier>, "wait for reply"=w300:bool)  [unwired: 1 out]
            n139 = Bundle By Name(cluster=T16 {"Module ID"=-1, "error"={"status"=FALSE, "code"=0, "source"=""}} ("Clear Motor Error (Reply Payload)"), "Module ID"=w296, "error"=w293) -> (w299:T16)
            n140 = Merge Errors(w305, w293) -> (w297:errorcluster)
            n141 = case "DQMH_FIRE_NOTIFIER" shown="True" w300 {
              tunnel: w301 -> [_ w311]
              tunnel: w299 -> [_ w310]
              frame False {
              }
              frame True {
                n142 = Send Notification(notification=w310, notifier=w311) -> ()  [unwired: 1 in, 2 out]
              }
            }
          }
          frame "read config" {
            n143 = Variant To Data(error in=w327, type=T8 {"Module ID"=-1, "config file path"=path "", "Wait Notifier"=refnum, "wait for reply"=FALSE} ("read config Argument"), Variant=w325) -> (data=w323:T8, error out=w326:errorcluster)
            n144 = property class="Mod Admin"(reference=w316) -> ("Accessors:Module ID"=w317:i32)  [unwired: 1 in, 2 out]
            n145 = Unbundle By Name(w323) -> ("config file path"=w314:path, "Wait Notifier"=w322:refnum<notifier>, "wait for reply"=w321:bool)  [unwired: 1 out]
            n146 = in-place {
              in-place-border: w314 -> [w329]
              in-place-border: [w328] -> w313
              n147 = in-place-cluster #4(w315) -> ("Stepper"=w331:refnum<class "Stepper.lvclass">)
              n148 = call-dynamic "read config.vi"("Config File Path"=w329, "Stepper in"=w331) -> ("error out"=w328:errorcluster, "Stepper out"=w330:refnum<class "Stepper.lvclass">)  [unwired: 8 in]
              n149 = in-place-cluster #4("Stepper"=w330) -> (w312:T2)
            }
            n150 = Bundle By Name(cluster=T17 {"Module ID"=-1, "error"={"status"=FALSE, "code"=0, "source"=""}} ("read config (Reply Payload)"), "Module ID"=w317, "error"=w313) -> (w320:T17)
            n151 = Merge Errors(w326, w313) -> (w318:errorcluster)
            n152 = case "DQMH_FIRE_NOTIFIER" shown="True" w321 {
              tunnel: w322 -> [_ w333]
              tunnel: w320 -> [_ w332]
              frame False {
              }
              frame True {
                n153 = Send Notification(notification=w332, notifier=w333) -> ()  [unwired: 1 in, 2 out]
              }
            }
          }
          frame "Read Angle" {
            n154 = Variant To Data(error in=w349, type=T9 {"Module ID"=-1, "Wait Notifier"=refnum, "wait for reply"=FALSE} ("Read Angle Argument"), Variant=w347) -> (data=w345:T9, error out=w348:errorcluster)
            n155 = property class="Mod Admin"(reference=w338) -> ("Accessors:Module ID"=w339:i32)  [unwired: 1 in, 2 out]
            n156 = Unbundle By Name(w345) -> ("Wait Notifier"=w344:refnum<notifier>, "wait for reply"=w343:bool)  [unwired: 1 out]
            n157 = in-place {
              in-place-border: [w351] -> w336
              in-place-border: [w350] -> w335
              n158 = in-place-cluster #5(w337) -> ("Stepper"=w353:refnum<class "Stepper.lvclass">)
              n159 = call-dynamic "read position.vi"("Stepper in"=w353) -> ("error out"=w350:errorcluster, "Angle"=w351:dbl, "Stepper out"=w352:refnum<class "Stepper.lvclass">)  [unwired: 8 in]
              n160 = in-place-cluster #5("Stepper"=w352) -> (w334:T2)
            }
            n161 = Bundle By Name(cluster=T18 {"Module ID"=-1, "Angle"=0.0, "error"={"status"=FALSE, "code"=0, "source"=""}} ("Read Angle (Reply Payload)"), "Module ID"=w339, "Angle"=w336, "error"=w335) -> (w342:T18)
            n162 = Merge Errors(w348, w335) -> (w340:errorcluster)
            n163 = case "DQMH_FIRE_NOTIFIER" shown="True" w343 {
              tunnel: w344 -> [_ w355]
              tunnel: w342 -> [_ w354]
              frame False {
              }
              frame True {
                n164 = Send Notification(notification=w354, notifier=w355) -> ()  [unwired: 1 in, 2 out]
              }
            }
          }
          frame "Jog" {
            n165 = property class="Mod Admin"(reference=w362) -> ("Accessors:Module ID"=w363:i32)  [unwired: 1 in, 2 out]
            n166 = Variant To Data(error in=w373, type=T10 {"Module ID"=-1, "CCW? (T)"=TRUE, "[rpm]"=60, "Wait Notifier"=refnum, "wait for reply"=FALSE} ("Jog Argument"), Variant=w371) -> (data=w369:T10, error out=w372:errorcluster)
            n167 = Unbundle By Name(w369) -> ("CCW? (T)"=w359:bool, "[rpm]"=w357:u16, "Wait Notifier"=w368:refnum<notifier>, "wait for reply"=w367:bool)  [unwired: 1 out]
            n168 = in-place {
              in-place-border: w359 -> [w382]
              in-place-border: [w379] -> w358
              in-place-border: [w378] -> w356
              in-place-border: w357 -> [w375]
              n169 = in-place-cluster #6(w361) -> ("Stepper"=w384:refnum<class "Stepper.lvclass">)
              n170 = call-dynamic "write single register.vi"("register to write"=w375, "address"=u16 481, "Stepper in"=w384) -> ("error out"=w376:errorcluster, "Stepper out"=w383:refnum<class "Stepper.lvclass">)  [unwired: 7 in]
              n171 = call-dynamic "jog motor.vi"("error in (no error)"=w376, "CCW? (T)"=w382, "Stepper in"=w383) -> ("error out"=w377:errorcluster, "Stepper out"=w381:refnum<class "Stepper.lvclass">)  [unwired: 7 in]
              n172 = call-dynamic "read position.vi"("error in (no error)"=w377, "Stepper in"=w381) -> ("error out"=w378:errorcluster, "Angle"=w379:dbl, "Stepper out"=w380:refnum<class "Stepper.lvclass">)  [unwired: 7 in]
              n173 = in-place-cluster #6("Stepper"=w380) -> (w360:T2)
            }
            n174 = Bundle By Name(cluster=T19 {"Module ID"=-1, "Angle"=0.0, "error"={"status"=FALSE, "code"=0, "source"=""}} ("Jog (Reply Payload)"), "Module ID"=w363, "Angle"=w358, "error"=w356) -> (w366:T19)
            n175 = Merge Errors(w372, w356) -> (w364:errorcluster)
            n176 = case "DQMH_FIRE_NOTIFIER" shown="True" w367 {
              tunnel: w368 -> [_ w386]
              tunnel: w366 -> [_ w385]
              frame False {
              }
              frame True {
                n177 = Send Notification(notification=w385, notifier=w386) -> ()  [unwired: 1 in, 2 out]
              }
            }
          }
          frame "Go To Angle" {
            n178 = Variant To Data(error in=w405, type=T11 {"Module ID"=-1, "Angle"=0.0, "Velocity [rpm]"=5, "Pause Time [ms]"=50, "Wait Notifier"=refnum, "wait for reply"=FALSE} ("Go To Angle Argument"), Variant=w403) -> (data=w401:T11, error out=w404:errorcluster)
            n179 = property class="Mod Admin"(reference=w394) -> ("Accessors:Module ID"=w395:i32)  [unwired: 1 in, 2 out]
            n180 = Unbundle By Name(w401) -> ("Angle"=w391:dbl, "Velocity [rpm]"=w390:i32, "Pause Time [ms]"=w389:i32, "Wait Notifier"=w400:refnum<notifier>, "wait for reply"=w399:bool)  [unwired: 1 out]
            n181 = in-place {
              in-place-border: w391 -> [w413]
              in-place-border: w390 -> [w412]
              in-place-border: w389 -> [w411]
              in-place-border: [w408] -> w388
              in-place-border: [w407] -> w387
              n182 = in-place-cluster #7(w393) -> ("Stepper"=w414:refnum<class "Stepper.lvclass">)
              n183 = call-dynamic "go to angle.vi"("Pause Time [ms]"=w411, "Velocity [rpm]"=w412, "Angle"=w413, "Stepper in"=w414) -> ("error out"=w406:errorcluster, "Stepper out"=w410:refnum<class "Stepper.lvclass">)  [unwired: 6 in]
              n184 = call-dynamic "read position.vi"("error in (no error)"=w406, "Stepper in"=w410) -> ("error out"=w407:errorcluster, "Angle"=w408:dbl, "Stepper out"=w409:refnum<class "Stepper.lvclass">)  [unwired: 7 in]
              n185 = in-place-cluster #7("Stepper"=w409) -> (w392:T2)
            }
            n186 = Bundle By Name(cluster=T20 {"Module ID"=-1, "Angle"=0.0, "error"={"status"=FALSE, "code"=0, "source"=""}} ("Go To Angle (Reply Payload)"), "Module ID"=w395, "Angle"=w388, "error"=w387) -> (w398:T20)
            n187 = Merge Errors(w404, w387) -> (w396:errorcluster)
            n188 = case "DQMH_FIRE_NOTIFIER" shown="True" w399 {
              tunnel: w400 -> [_ w416]
              tunnel: w398 -> [_ w415]
              frame False {
              }
              frame True {
                n189 = Send Notification(notification=w415, notifier=w416) -> ()  [unwired: 1 in, 2 out]
              }
            }
          }
          frame "---Copy This Frame---" {
            # "Duplicate this frame when creating new messages.  Change this comment in the duplicated frame to describe this message."
            n190 = Merge Errors(w419) -> (w418:errorcluster)
          }
          frame "---Exit and Error Handling---" {
            # "Separator - the following cases handle errors and exit messages."
          }
          frame "Error" {
            # "#DQMH_CodeRecommended - If the module is running in standalone mode (External Launch = FALSE), this code will pop up an error dialog and call the 'Exit' message if an error occurs. Add more fine-grained error management here."
            # "Error - Check the error message data and respond accordingly. This message is sent by the \"Error Handler\" VIs at the end of each loop in this application."
            n191 = property on="Property Node" class="Mod Admin"(reference=w426) -> ("Accessors:External Launch"=w425:bool, "Accessors:Module ID"=w423:i32)  [unwired: 1 in, 2 out]
            n192 = Variant To Data(error in=w433, type=errorcluster {"status"=FALSE, "code"=0, "source"=""} ("error constant"), Variant=w427) -> (data=w422:errorcluster, error out=w431:errorcluster)
            n193 = local write "error out"(w422) -> ()
            n194 = call "Error Reported.vi"("Error"=w422, "Module ID"=w423) -> ()  [unwired: 9 in, 1 out]
            n195 = case shown="False" w425 {
              tunnel: [w438 _] -> w430
              tunnel: w424 -> [w436 _]
              tunnel: w422 -> [w437 _]
              frame False {
                n196 = disable-structure shown="Default" {
                  disable-tunnel: w437 -> [w439 _]
                  frame condition #0 (active) {
                    # "If the module is running standalone, then pop up an error dialog and call the \"Exit\" message."
                    n197 = call <vilib>:"Simple Error Handler.vi"("error in (no error)"=w439) -> ()  [unwired: 4 in, 5 out]
                  }
                  frame condition #1 {
                    # "To prevent the Simple Error Handler VI from being loaded (e.g. when deploying to a Real-Time target), add the Conditional Disable Symbol \"DQMH_Disable_SEH\" to your project and set it to TRUE."
                  }
                }
                n198 = call-poly <vilib>:"Delacor_lib_QMH_Enqueue Message (poly).vi"("Priority Message? (F)"=TRUE, "Message"="Exit", "Message Queue in"=w436) -> ("error out"=w438:errorcluster)  [unwired: 7 in, 1 out]
              }
              frame True {
                # "If the module was launched externally, calling the Error Reported broadcast VI is the only action performed by the \"Error\" message. The module's caller can then process the error appropriately."
              }
            }
            n199 = Merge Errors(w431, w430) -> (w429:errorcluster)
          }
          frame "Simulate MHL Error" {
            # "#DQMH_HowTo The 'Simulate MHL Error' button  illustrates how the MHL handles errors. This event is instructional in nature and can be removed."
            # "Simulate an error occurring at the MHL"
            n200 = property on="Property Node" class="Mod Admin"(reference=w445) -> ("Accessors:Module ID"=w446:i32)  [unwired: 1 in, 2 out]
            n201 = call "Module Name--constant.vi"("Module ID"=w446) -> ("Module Name"=w441:string)  [unwired: 10 in]
            n202 = Format Into String(format string="Simulated error originating at Message Handling Loop in %s", w441) -> (resulting string=w442:string)  [unwired: 2 in, 1 out]
            n203 = call <vilib>:"Error Cluster From Error Code.vi"("show call chain? (False)"=TRUE, "error message (\"\")"=w442, "error code (0)"=5001) -> ("error out"=w448:errorcluster)  [unwired: 6 in]
            n204 = Merge Errors(w450, w448) -> (w449:errorcluster)
          }
          frame "Exit" {
            w458 = 91  # 91: not all Exit messages will have an argument
            w459 = TRUE  # Stop the VI
            # "Release the message queue reference"
            # "#DQMH_CodeNeeded - Add any required cleanup code here."
            # "Exit - Exit the application."
            n205 = Variant To Data(error in=w467, type=T4 {"Module ID"=-1, "Origin"="", "Exit via Stop Module Req?"=FALSE, "Wait for Module to stop?"=FALSE} ("Stop Argument"), Variant=w457) -> (data=w454:T4, error out=w463:errorcluster)
            n206 = call <vilib>:"Clear Errors.vi"("error in (no error)"=w463, "specific error code to clear (0: all)"=w458) -> ("error out"=w466:errorcluster)  [unwired: 4 in, 1 out]
            n207 = property on="Property Node" class="Mod Admin"(reference=w452) -> ("Accessors:Module ID"=w451:i32)  [unwired: 1 in, 2 out]
            n208 = control-ref of="This VI"() -> (w453:refnum<vi>)
            n209 = call-dynamic "Delacor_lib_QMH_Release Message Queue.vi"("error in"=w466, "Message Queue"=w461) -> ("error out"=w465:errorcluster)  [unwired: 9 in]
            n210 = call "Handle Exit.vi"("Stop Argument"=w454, "Module Admin in"=w452, "VI reference"=w453) -> ("error out"=w464:errorcluster, "Wait for Stop?"=w455:bool)  [unwired: 7 in]
            n211 = Merge Errors(w465, w464) -> (w462:errorcluster)
            n212 = call "Error Reported.vi"("Error"=w462, "Module ID"=w451) -> ()  [unwired: 9 in, 1 out]
          }
          frame Default {
            # "'Default' case only runs if there is a message that isn't defined in any of the other cases.  Output a programming error."
            n213 = property on="Property Node" class="Mod Admin"(reference=w475) -> ("Accessors:Module ID"=w474:i32)  [unwired: 1 in, 2 out]
            n214 = call "Module Name--constant.vi"("Module ID"=w474) -> ("Module Name"=w468:string)  [unwired: 10 in]
            n215 = Format Into String(format string="The invalid message string \"%s\" was received in the Message Handling Loop for module \"%s\".", w469, w468) -> (resulting string=w471:string)  [unwired: 2 in, 1 out]
            n216 = call <vilib>:"Error Cluster From Error Code.vi"("show call chain? (False)"=TRUE, "error message (\"\")"=w471, "error code (0)"=1) -> ("error out"=w477:errorcluster)  [unwired: 6 in]
            n217 = Merge Errors(w478, w477) -> (w479:errorcluster)
          }
        }
        n218 = call-dynamic "Delacor_lib_QMH_Error Handler - Message Handling Loop.vi"("error in"=w228, "Message Queue in"=w219) -> ("dup error in"=w225:errorcluster)  [unwired: 8 in, 1 out]
      }
    }
    frame Error {
      n219 = call "Synchronize Caller Events.vi"("Module Admin"=w483) -> ("Module Admin out"=w482:refnum<class "Delacor_lib_QMH_Cloneable Module Admin.lvclass">)  [unwired: 9 in, 1 out]
      n220 = property on="Property Node" class="Mod Admin"(reference=w482) -> ("Accessors:Module ID"=w481:i32)  [unwired: 1 in, 2 out]
      n221 = call-dynamic "Delacor_lib_QMH_Release Message Queue.vi"("error in"=w489, "Message Queue"=w480) -> ("error out"=w488:errorcluster)  [unwired: 9 in]
      n222 = call "Module Name--constant.vi"("Module ID"=w481) -> ("Module Name"=w486:string)  [unwired: 10 in]
      n223 = Format Into String(format string="An error occurred during initialization. %s is no longer running.", w486) -> (resulting string=w484:string)  [unwired: 2 in, 1 out]
      n224 = call "Error Reported.vi"("Additional Information"=w484, "Error"=w488, "Module ID"=w481) -> ()  [unwired: 8 in, 1 out]
    }
  }
  n225 = Merge Errors(w17, w16) -> (w18:errorcluster)
  n226 = call "Close Module.vi"("error in"=w18, "Wait for stop?"=w2, "Module Admin in"=w4) -> ("error out"=w14:errorcluster, "External Launch"=w1:bool, "Module Admin out"=w3:refnum<class "Delacor_lib_QMH_Cloneable Module Admin.lvclass">)  [unwired: 6 in]
  n227 = Unregister For Events(event registration refnum=w9, error in=w14) -> (error out=w13:errorcluster)
  "error out" <- w13
  n228 = case "External Launch?" shown="True" w1 {
    tunnel: w13 -> [_ w490]
    frame False {
    }
    frame True {
      n229 = case shown="No Error" w490 {
        frame No Error {
          n230 = invoke class="VI" method="FP.Close"() -> ()  [unwired: 3 in, 3 out]
        }
        frame Error {
          n231 = disable-structure shown="Default" {
            frame condition #0 (active) {
              n232 = invoke class="VI" method="FP.Open"("Activate"=TRUE ("Activate?")) -> ()  [unwired: 4 in, 5 out]
            }
            frame condition #1 {
              # "Don't show panel on error if running inside a built EXE."
            }
          }
        }
      }
    }
  }
  n233 = local write "Module Admin"(w3) -> ()
